vi "Configure Dialog.vi"(8 "Error In":errorcluster, 11 "Quench Msg in":refnum<class "Quench Msg.lvclass">) -> (0 "Error Out":errorcluster, 2 "OK?":bool, 3 "Quench Msg out":refnum<class "Quench Msg.lvclass">)   [LabVIEW 2016, in "KIT-QVA.lvlib" / "Quench Msg.lvclass"]
doc: "This overrides of this dynamic dispatch VI open the frontpanel to set derived message attributes."
uses:
  Quench Msg.lvclass
  Quench Msg.lvclass/Quench Msg.ctl
panel:
  in  "Quench":bool
  in  "OK":bool
  in  "Cancel":bool
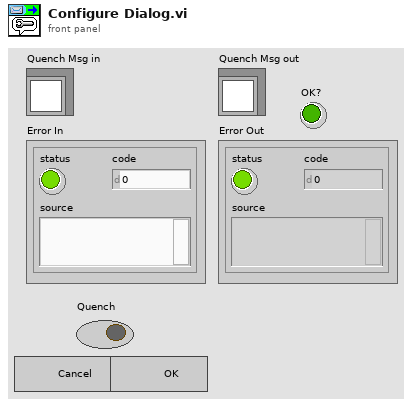
[diagram p1: front panel]
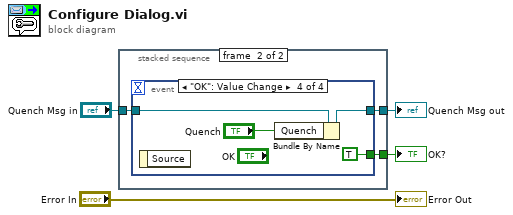
[diagram p0: block diagram]
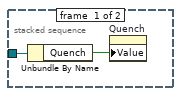
[diagram p2: hidden frame]
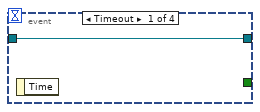
[diagram p3: hidden frame]
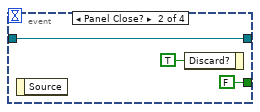
[diagram p4: hidden frame]
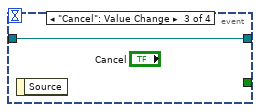
[diagram p5: hidden frame]
diagram:
  n1 = stacked-sequence {
    tunnel: "Quench Msg in" -> [w6 w9]
    tunnel: [_ w8] -> w2
    tunnel: [_ w7] -> w1
    frame #0 {
      n2 = Unbundle By Name(w6) -> ("Quench"=w5:bool)
      n3 = property on="Quench" class="Bool (strict)"("Value"=w5) -> ()  [unwired: 2 in, 2 out]
    }
    frame #1 {
      n4 = event shown="[3] \"OK\": Value Change" {
        selector: _ -> [_ _ _ _]
        dyn-events: _ -> [_ _ _ _]
        timeout: _ -> [_ _ _ _]
        tunnel: [w10 w11 w14 w17] -> w7
        tunnel: w9 -> [w10 w11 w14 w18]
        tunnel: [_ FALSE _ TRUE] -> w8
        event Timeout {
          n5 = event-data() -> ()  [unwired: 1 in, 1 out]
        }
        event Panel Close? {
          n6 = event-data() -> ()  [unwired: 1 in, 1 out]
          n7 = event-data("Discard?"=TRUE) -> ()  [unwired: 1 in, 1 out]
        }
        event "Cancel": Value Change {
          n8 = event-data() -> ()  [unwired: 1 in, 1 out]
        }
        event "OK": Value Change {
          n9 = event-data() -> ()  [unwired: 1 in, 1 out]
          n10 = Bundle By Name(cluster=w18, "Quench"="Quench") -> (w17:refnum<class "Quench Msg.lvclass">)
        }
      }
    }
  }
  "Quench Msg out" <- w1
  "OK?" <- w2
  "Error Out" <- "Error In"
